vi "K-L transform.vi"(0 "Dataset":dbl[][](array[numeric])) -> (1 "Final Dataset":dbl[](array[numeric]), 2 "Eigenvalues":cdb[](array[numeric]), 3 "Feature Vector":dbl[](array[numeric]), 4 "Eigenvectors":T2)   [LabVIEW 2013]
uses:
  <vilib>/Analysis/Matrix/Datatypes/ComplexMatrix.ctl
  <vilib>/Analysis/Matrix/Datatypes/RealMatrix.ctl
  <vilib>/Analysis/Matrix/Numeric/Conversions/Array To Matrix - RA2.vi
  <vilib>/Analysis/7linalg.llb/Real Eigenvalues and Vectors.vi
  <vilib>/Analysis/Matrix/Numeric/Complex/Complex To Polar - CM.vi
  <vilib>/Analysis/Matrix/Numeric/Multiply/Multiply - RM,RM.vi
  <vilib>/Analysis/Matrix/Numeric/Conversions/Matrix To Array - RM.vi
  <vilib>/gmath/NI_Gmath.lvlib
  <vilib>/Analysis/NI_AALPro.lvlib
  <vilib>/Analysis/Matrix/NI_Matrix.lvlib
panel:
  out "theta":dbl[](array[numeric])
  out "max index(es)":i32
  out "covariance matrix V":T1
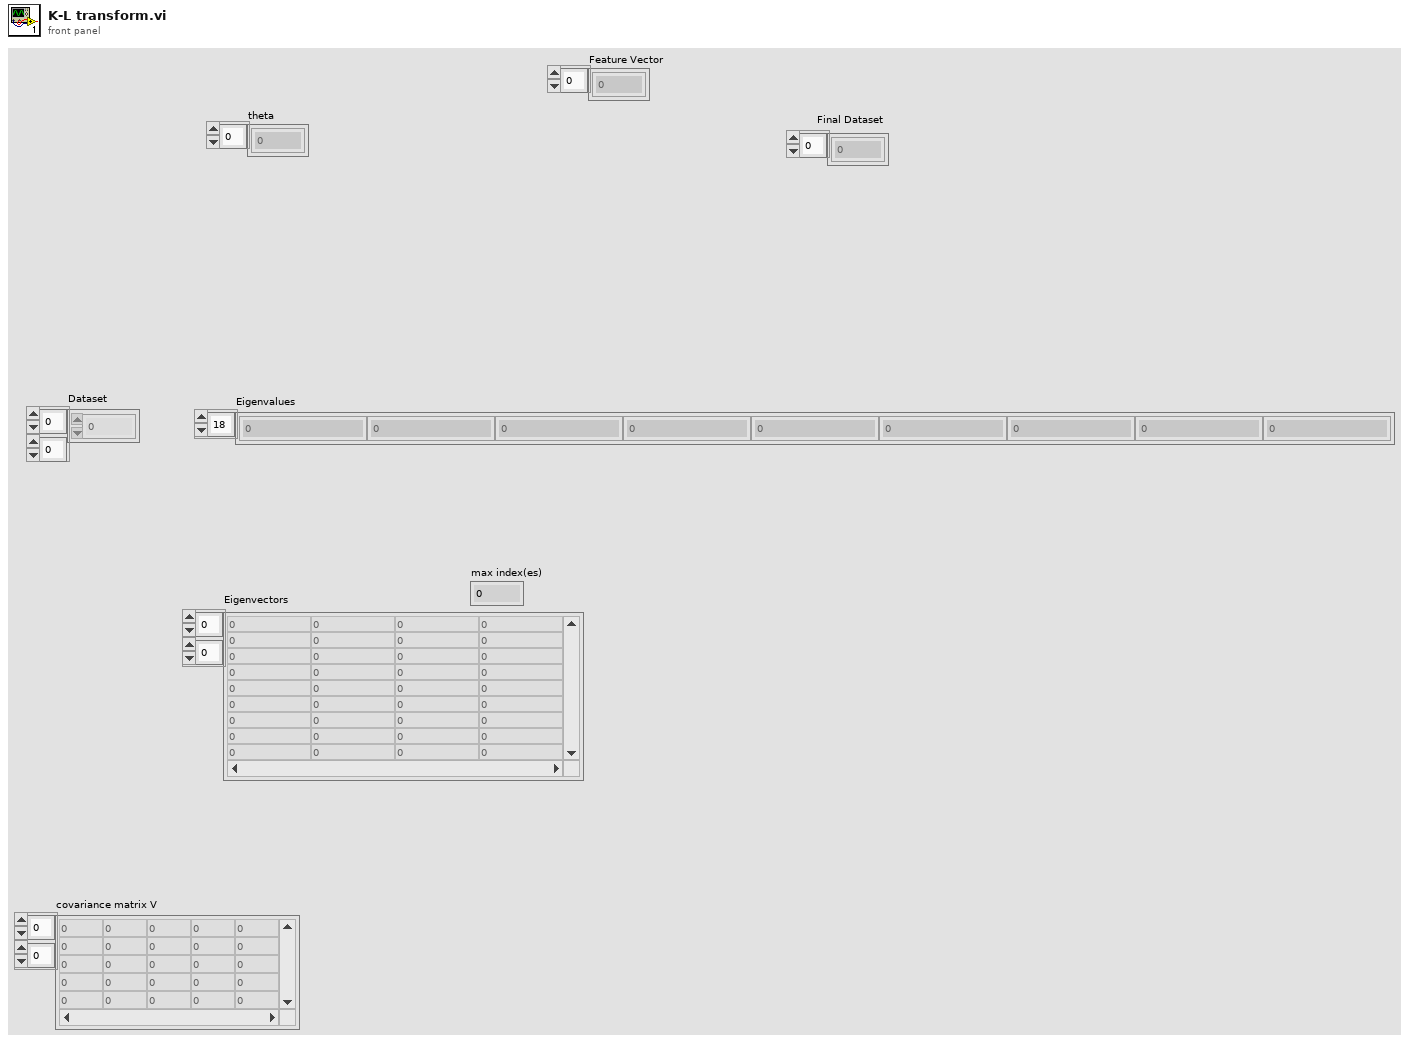
[diagram p1: front panel]
types:
  T1 = typedef "NI_Matrix.lvlib/RealMatrix.ctl" = dbl[][]
  T2 = typedef "NI_Matrix.lvlib/ComplexMatrix.ctl" = cdb[][]
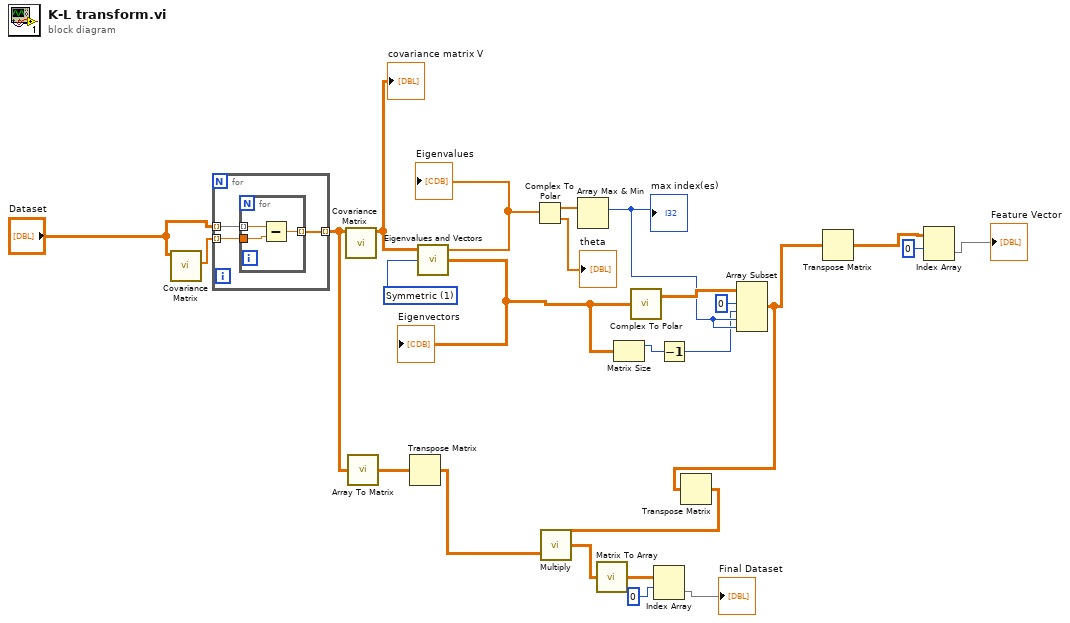
[diagram p0: block diagram]
diagram:
  w23 = 1 items=["General", "Symmetric"] ("matrix type")
  n1 = call <vilib>:"Covariance Matrix.vi"("X"="Dataset") -> ("mean vector"=w25:dbl[])  [unwired: 9 in, 1 out]
  n2 = for {
    tunnel: "Dataset" -> [w28] mode=indexing
    tunnel: w25 -> [w27] mode=indexing
    tunnel: [w26] -> w12 mode=indexing
    n3 = for {
      tunnel: w28 -> [w31] mode=indexing
      tunnel: w27 -> [w30]
      tunnel: [w29] -> w26 mode=indexing
      n4 = Subtract(x=w31, y=w30) -> (x-y=w29:dbl)
    }
  }
  n5 = call <vilib>:"Covariance Matrix.vi"("X"=w12) -> ("covariance matrix V"=w24:T1)  [unwired: 9 in, 1 out]
  "covariance matrix V" <- w24
  n6 = call-poly <vilib>:"Array To Matrix.vi"("Real 2D Array"=w12) -> ("Real Matrix"=w14:T1)
  n7 = Transpose Matrix(1:w14) -> (0:w10:T1)
  n8 = call-poly <vilib>:"Eigenvalues and Vectors.vi"("matrix type"=w23, "Input Matrix"=w24) -> ("Eigenvectors"=w19:T2, "Eigenvalues"=w21:cdb[])  [unwired: 1 in, 1 out]
  "Eigenvalues" <- w21
  "Eigenvectors" <- w19
  n9 = Complex To Polar(r * e^(i*theta)=w21) -> (r=w22:dbl[], theta=→"theta":dbl[])
  n10 = Array Max & Min(array=w22) -> (max index (indices)=w16:i32)  [unwired: 3 out]
  "max index(es)" <- w16
  n11 = Matrix Size(0:w19) -> (1:w15:i32)  [unwired: 1 out]
  n12 = call-poly <vilib>:"Complex To Polar.vi"("Complex Matrix r*e^iQ"=w19) -> ("Modulus r"=w18:T1)  [unwired: 1 out]
  n13 = Decrement(x=w15) -> (x-1=w6:i32)
  n14 = Array Subset(array=w18, index (row)=0 ("row 1"), length (row)=w6, index (col)=w16, length (col)=w16) -> (w3:T1)
  n15 = Transpose Matrix(1:w3) -> (0:w11:T1)
  n16 = call-poly <vilib>:"Multiply.vi"("Real Matrix B"=w10, "Real Matrix A"=w11) -> ("A * B"=w9:T1)
  n17 = call-poly <vilib>:"Matrix To Array.vi"("Real Matrix"=w9) -> ("Real 2D Array"=w8:dbl[][])
  n18 = Index Array(array=w8, index (row)=0 ("index")) -> (element=→"Final Dataset":dbl[])  [unwired: 1 in]
  n19 = Transpose Matrix(1:w3) -> (0:w2:T1)
  n20 = Index Array(array=w2, index (row)=0 ("index")) -> (element=→"Feature Vector":dbl[])  [unwired: 1 in]
